vi "rs3 Advanced get census diameter3.vi"(8 "error in (no error)":errorcluster, 10 "mode":i32, 11 "device in":u64) -> (0 "error out 2":errorcluster, 1 "error":u64, 2 "ST_CensusEnable":cluster{"uDiameter":u32, "vDiameter":u32}={"uDiameter"=15, "vDiameter"=15}, 3 "Dev out":u64)   [LabVIEW 2017, in "libRealSense3.lvlib"]
doc: "Opens communication to a specific RealSense Device."
uses:
  libRealSense3.lvlib
  realsense2.dll
panel:
  # "RS3 Adv. Get Census diameter"
  # "(C) 2017 Intel Corp.,  AGJ"
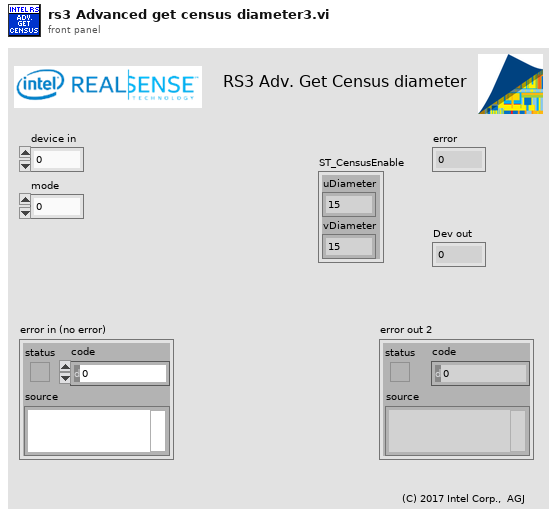
[diagram p1: front panel]
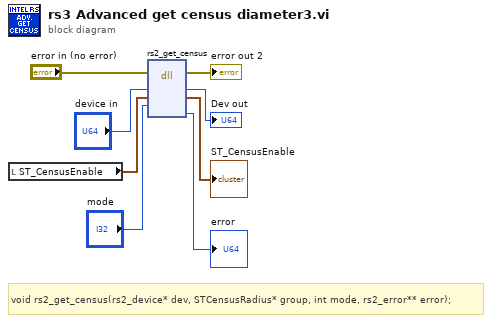
[diagram p0: block diagram]
diagram:
  # "void rs2_get_census(rs2_device* dev, STCensusRadius* group, int mode, rs2_error** error);"
  n1 = local read "ST_CensusEnable"() -> (w3:cluster{"uDiameter":u32, "vDiameter":u32})
  n2 = dll-call lib="C:/Users/agrunnet/Documents/libRealSense6/realsense2.dll" fn="rs2_get_census"(error in="error in (no error)", "device"="device in", "census"=w3, "mode"="mode") -> (error out=→"error out 2":errorcluster, "device"=→"Dev out":u64, "census"=→"ST_CensusEnable":cluster{"uDiameter":u32, "vDiameter":u32}, "error"=→"error":u64)  [unwired: 5 in, 1 out]
